vi "Sigma_GetPos.vi"(0 "VISA resource name":refnum<visa-resource-name>, 5 "Travel per Pulse (mm)":dbl=0.004, 7 "Init Pos X (mm)":dbl format="%#_4g", 9 "Init  Pos Y (mm)":dbl format="%#_4g", 11 "error in (no error)":errorcluster) -> (2 "Pos X (mm)":dbl format="%#_4g", 3 "Pos Y (mm)":dbl format="%#_4g", 4 "VISA resource name out":refnum<visa-resource-name>, 10 "State String":string, 15 "error out":errorcluster)   [LabVIEW 2018]
panel:
  out "길이":i32
  out "숫자형":i32
  out "read buffer":string
  out "Serial Settings:Number of Bytes at Serial Port":u32
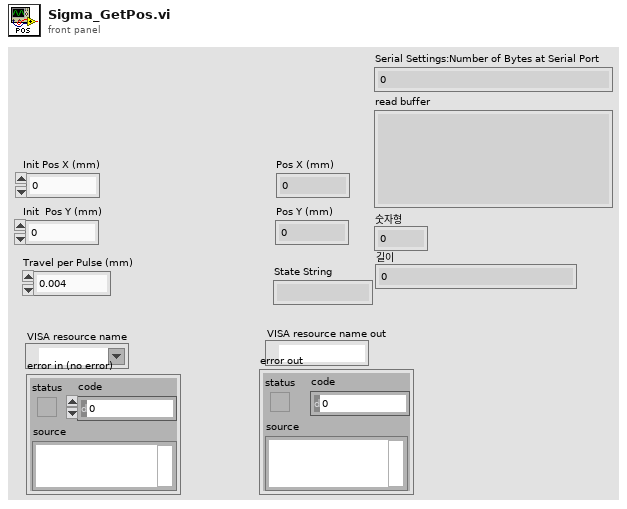
[diagram p1: front panel]
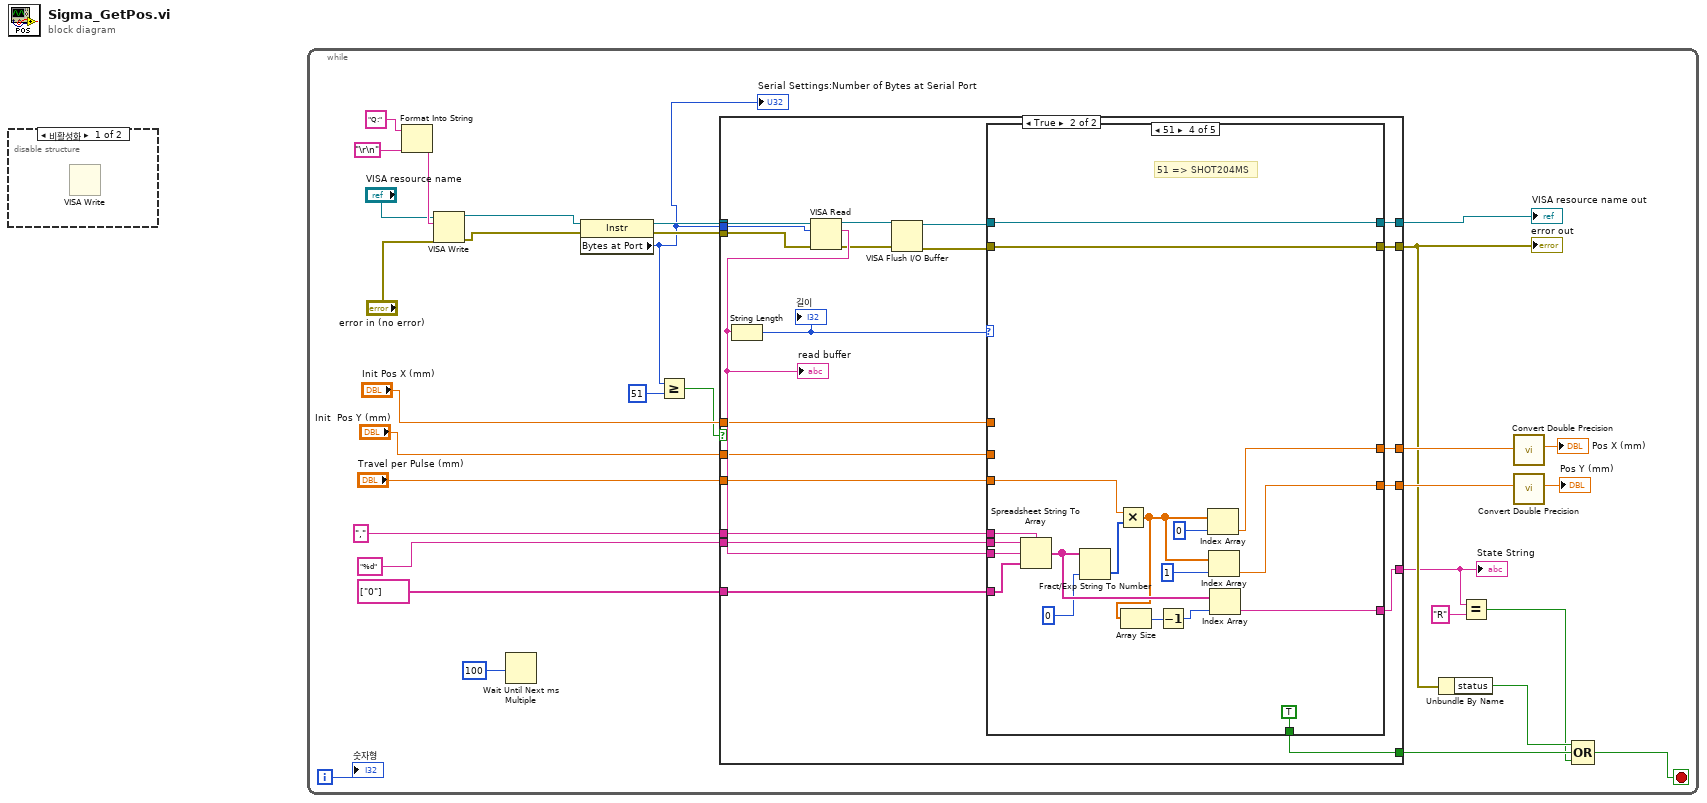
[diagram p0: block diagram]
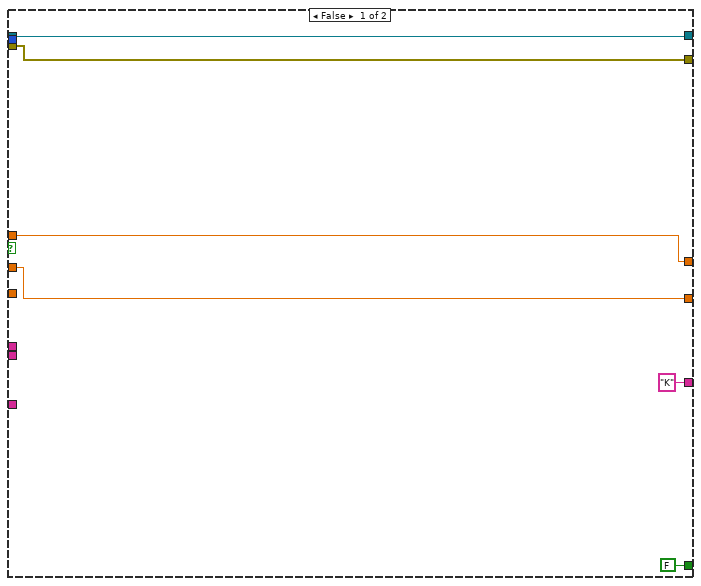
[diagram p3: hidden frame]
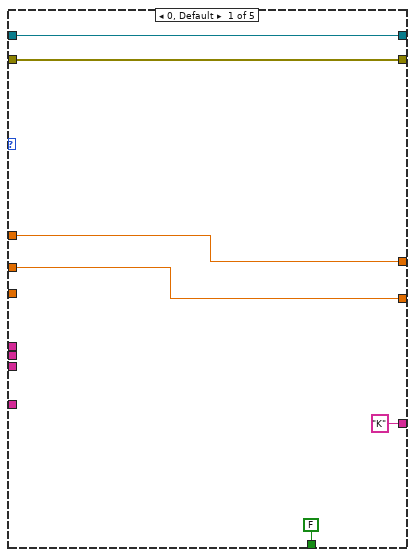
[diagram p4: hidden frame]
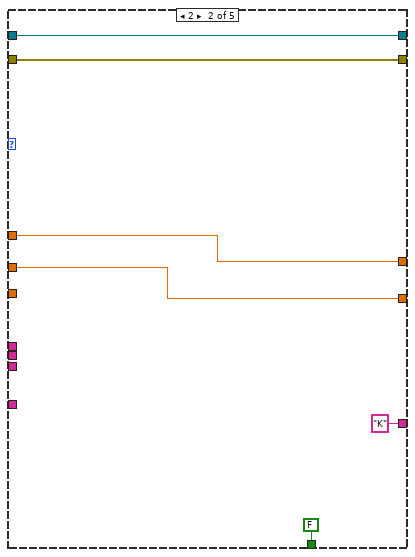
[diagram p5: hidden frame]
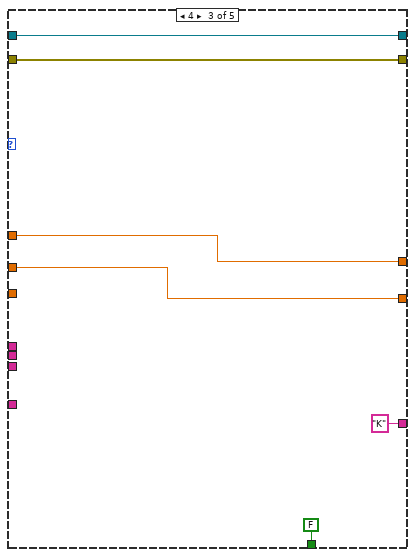
[diagram p6: hidden frame]
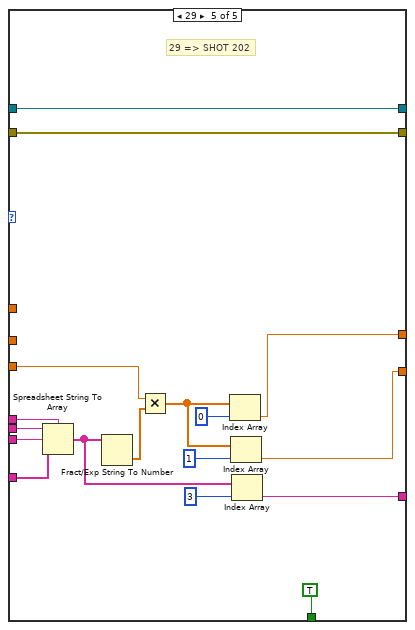
[diagram p7: hidden frame]
diagram:
  n1 = disable-structure shown="비활성화" {
    frame Disabled {
      n2 = VISA Write() -> ()  [unwired: 3 in, 3 out]
    }
    frame Enabled {
    }
  }
  n3 = while {
    i -> [w13]
    stop <- w15 stop-if-true
    n4 = Format Into String(initial string="Q:" ("string"), "\r\n") -> (resulting string=w8:string)  [unwired: 2 in, 1 out]
    n5 = VISA Write(VISA resource name="VISA resource name", write buffer=w8, error in (no error)="error in (no error)") -> (VISA resource name out=w3:refnum<visa-resource-name>, error out=w2:errorcluster)  [unwired: 1 out]
    n6 = Wait Until Next ms Multiple(millisecond multiple=u32 100 ("milliseconds to wait")) -> ()  [unwired: 1 out]
    n7 = property class="Instr"(reference=w3, error in=w2) -> (reference out=w28:refnum<visa-resource-name>, error out=w27:errorcluster, "Bytes at Port"=w7:u32)
    "Serial Settings:Number of Bytes at Serial Port" <- w7
    n8 = Greater Or Equal?(x=w7, y=u32 51) -> (x >= y?=w1:bool)
    n9 = case shown="True" w1 {
      tunnel: "," ("delimiter (Tab)") -> [_ w59]
      tunnel: "%d" ("format string") -> [_ w58]
      tunnel: string[] ["0"] ("Array") -> [_ w57]
      tunnel: "Travel per Pulse (mm)" -> [_ w56]
      tunnel: w28 -> [w38 w55]
      tunnel: w27 -> [w37 w54]
      tunnel: "Init  Pos Y (mm)" -> [w35 w51]
      tunnel: "Init Pos X (mm)" -> [w36 w50]
      tunnel: [w38 w49] -> w22
      tunnel: [w36 w48] -> w21
      tunnel: [w35 w47] -> w19
      tunnel: [w37 w46] -> w17
      tunnel: [FALSE ("status") w45] -> w14
      tunnel: w7 -> [_ w44]
      tunnel: ["K" ("String") w43] -> w12
      frame False {
      }
      frame True {
        n10 = VISA Read(VISA resource name=w55, byte count=w44, error in (no error)=w54) -> (VISA resource name out=w42:refnum<visa-resource-name>, read buffer=w52:string, error out=w41:errorcluster)  [unwired: 1 out]
        "read buffer" <- w52
        n11 = String Length(string=w52) -> (length=w53:i32)
        "길이" <- w53
        n12 = VISA Flush I/O Buffer(VISA resource name=w42, error in (no error)=w41) -> (VISA resource name out=w40:refnum<visa-resource-name>, error out=w39:errorcluster)  [unwired: 1 in]
        n13 = case shown="51" w53 {
          tunnel: w59 -> [_ _ _ w94 w111]
          tunnel: w58 -> [_ _ _ w93 w110]
          tunnel: w57 -> [_ _ _ w82 w109]
          tunnel: w56 -> [_ _ _ w90 w105]
          tunnel: w52 -> [_ _ _ w89 w104]
          tunnel: [w65 w70 w76 w88 w103] -> w48
          tunnel: [w64 w71 w77 w87 w102] -> w47
          tunnel: ["K" ("String") "K" ("String") "K" ("String") w86 w101] -> w43
          tunnel: w51 -> [w64 w71 w77 _ _]
          tunnel: w50 -> [w65 w70 w76 _ _]
          tunnel: [w62 w68 w74 w85 w100] -> w49
          tunnel: w40 -> [w62 w68 w74 w85 w100]
          tunnel: [w61 w67 w73 w84 w99] -> w46
          tunnel: w39 -> [w61 w67 w73 w84 w99]
          tunnel: [FALSE ("status") FALSE ("status") FALSE ("status") TRUE ("status") TRUE ("status")] -> w45
          frame 0, Default {
          }
          frame 2 {
          }
          frame 4 {
          }
          frame 51 {
            # "51 => SHOT204MS"
            n14 = Spreadsheet String To Array(delimiter (Tab)=w94, format string=w93, spreadsheet string=w89, array type (2D Dbl)=w82) -> (array=w92:string[])
            n15 = Fract/Exp String To Number(string=w92, default (0 dbl)=0) -> (number=w91:i32[])  [unwired: 2 in, 1 out]
            n16 = Multiply(x=w90, y=w91) -> (x*y=w81:dbl[])
            n17 = Array Size(array=w81) -> (size(s)=w80:i32)
            n18 = Decrement(x=w80) -> (x-1=w79:i32)
            n19 = Index Array(array=w81, index=0) -> (element=w88:dbl)
            n20 = Index Array(array=w81, index=1) -> (element=w87:dbl)
            n21 = Index Array(array=w92, index=w79) -> (element=w86:string)
          }
          frame 29 {
            # "29 => SHOT 202"
            n22 = Spreadsheet String To Array(delimiter (Tab)=w111, format string=w110, spreadsheet string=w104, array type (2D Dbl)=w109) -> (array=w107:string[])
            n23 = Fract/Exp String To Number(string=w107) -> (number=w106:dbl[])  [unwired: 3 in, 1 out]
            n24 = Multiply(x=w105, y=w106) -> (x*y=w98:dbl[])
            n25 = Index Array(array=w98, index=0) -> (element=w103:dbl)
            n26 = Index Array(array=w98, index=1) -> (element=w102:dbl)
            n27 = Index Array(array=w107, index=3) -> (element=w101:string)
          }
        }
      }
    }
    "VISA resource name out" <- w22
    "error out" <- w17
    "State String" <- w12
    n28 = Unbundle By Name(w17) -> ("status"=w16:bool)
    n29 = Equal?(x=w12, y="R") -> (x = y?=w10:bool)
    n30 = call "Convert Double Precision.vi"("Input"=w21) -> ("Output"=→"Pos X (mm)":dbl)  [unwired: 10 in]
    n31 = call "Convert Double Precision.vi"("Input"=w19) -> ("Output"=→"Pos Y (mm)":dbl)  [unwired: 10 in]
    n32 = Compound Arithmetic op=OR(w16, w14, w10) -> (w15:bool)
    "숫자형" <- w13
  }
